vi "Read Record Data.vi"(8 "Error In (no error)":errorcluster, 11 "Expenses Tracker Record In":refnum<class "Expenses Tracker Record.lvclass">) -> (0 "Error Out":errorcluster, 2 "Record":variant, 3 "Expenses Tracker Record Out":refnum<class "Expenses Tracker Record.lvclass">)   [LabVIEW 2023, in "Expenses Tracker Record.lvclass"]
uses:
  Expenses Tracker Record.lvclass
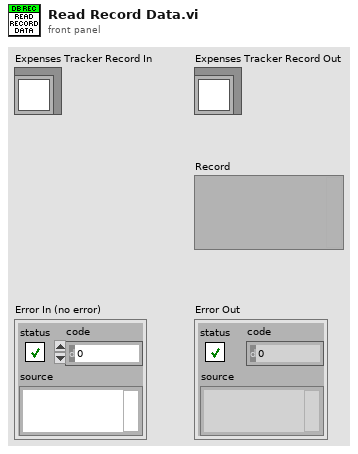
[diagram p1: front panel]
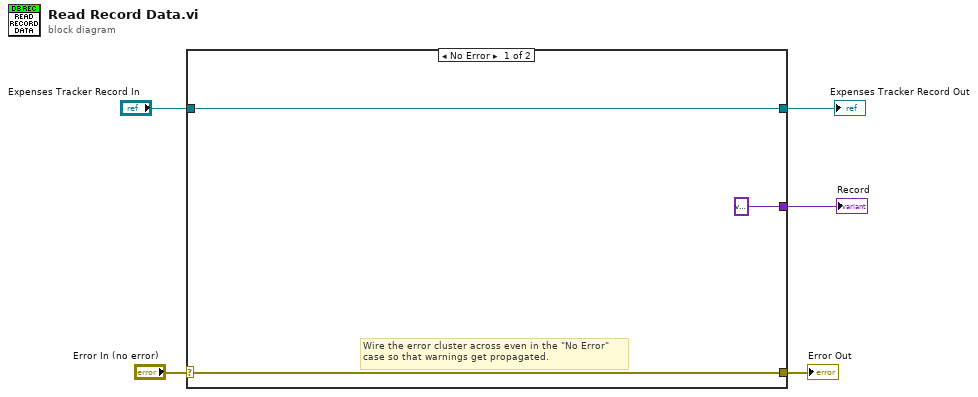
[diagram p0: block diagram]
diagram:
  n1 = case shown="No Error" "Error In (no error)" {
    selector: "Error In (no error)" -> [w7 w10]
    tunnel: [w7 w10] -> w4
    tunnel: [w8 w9] -> w1
    tunnel: "Expenses Tracker Record In" -> [w8 w9]
    tunnel: [variant _] -> w3
    frame No Error {
      # "Wire the error cluster across even in the \"No Error\"\ncase so that warnings get propagated."
    }
    frame Error {
    }
  }
  "Error Out" <- w4
  "Record" <- w3
  "Expenses Tracker Record Out" <- w1
